vi "Build Report String.vi"(8 "error in (no error)":errorcluster, 10 "Report Data":T1, 11 "Image Assertion in":refnum<class "Image Assertion.lvclass">) -> (0 "error out":errorcluster, 2 "Report String":string, 3 "Image Assertion out":refnum<class "Image Assertion.lvclass">)   [LabVIEW 2020, in "MacroAssert.lvlib" / "Image Assertion.lvclass"]
doc: "Builds a string using <B>Step</B> and <B>Report Data</B> to be included in a report."
uses:
  Image Assertion.lvclass
  Image Assertion.lvclass/Image Assertion.ctl
  MacroAssert.lvlib
  CTLs/Report Data.ctl
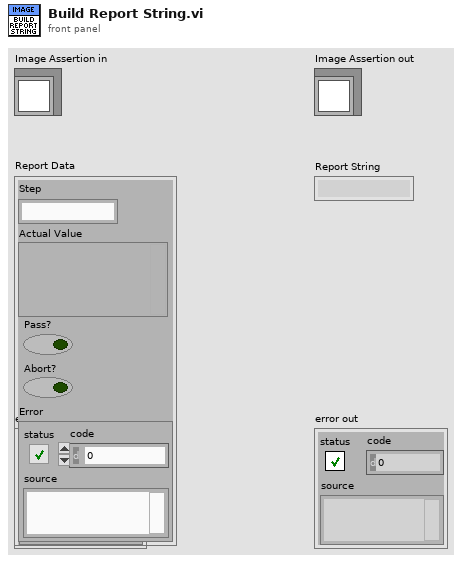
[diagram p1: front panel]
types:
  T1 = typedef "MacroAssert.lvlib/Report Data.ctl" = cluster{"Step":string, "Actual Value":variant, "Pass?":bool, "Abort?":bool, "Error":errorcluster}
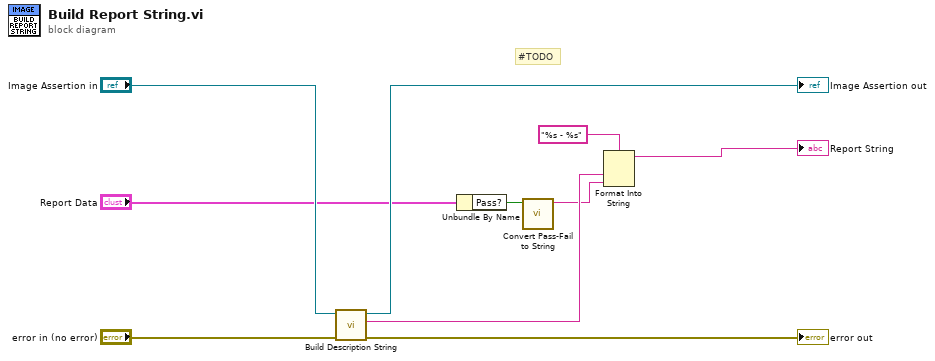
[diagram p0: block diagram]
diagram:
  # "#TODO"
  n1 = call-dynamic "Build Description String.vi"("error in (no error)"="error in (no error)", "Image Assertion in"="Image Assertion in") -> ("error out"=→"error out":errorcluster, "Description"=w9:string, "Image Assertion out"=→"Image Assertion out":refnum<class "Image Assertion.lvclass">)  [unwired: 7 in]
  n2 = Unbundle By Name("Report Data") -> ("Pass?"=w7:bool)
  n3 = call "Convert Pass-Fail to String.vi"("Pass?"=w7) -> ("Pass/Fail String"=w8:string)  [unwired: 10 in]
  n4 = Format Into String(format string="%s - %s", w9, w8) -> (resulting string=→"Report String":string)  [unwired: 2 in, 1 out]
